vi "getPathName.vi"(2 "error in":errorcluster, 3 "No.":i32) -> (0 "error out":errorcluster, 1 "resulting string":string)   [LabVIEW 2014]
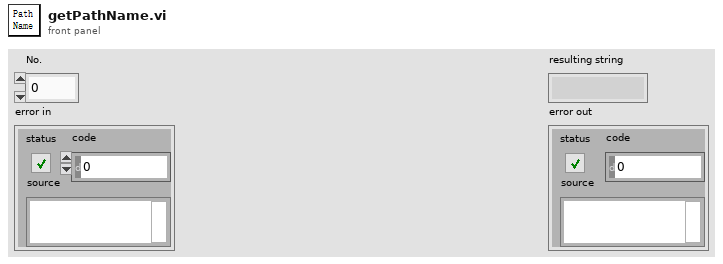
[diagram p1: front panel]
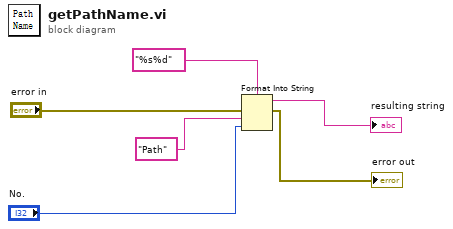
[diagram p0: block diagram]
diagram:
  n1 = Format Into String(format string="%s%d", error in="error in", "Path" ("input 1"), "No.") -> (resulting string=→"resulting string":string, error out=→"error out":errorcluster)  [unwired: 1 in]
